vi "test26-MappingRelationshipByLocalRegistration_WithSubcriberName.vi"(8 "error in (no error)":errorcluster, 11 "TestCase in":refnum<class "testcase-CSMBroadcast.lvclass">) -> (0 "error out":errorcluster, 3 "TestCase out":refnum<class "testcase-CSMBroadcast.lvclass">)   [LabVIEW 2017, in "testcase-CSMBroadcast.lvclass"]
uses:
  testcase-CSMBroadcast.lvclass
  caa41fc0-4920-4570-a7eb-0567c3b7bd6c.vi
  <vilib>/addons/_JKI Toolkits/VI Tester/TestCase.llb/TestCase.lvclass
  src/user.lib/_NEVSTOP/Communicable State Machine(CSM)/Communicable State Machine.lvlib
  C:/Program Files (x86)/National Instruments/LabVIEW 2017/vi.lib/addons/_JKI Toolkits/VI Tester/TestCase.llb/TestCase.lvclass
panel:
  out "Loop Count":i32
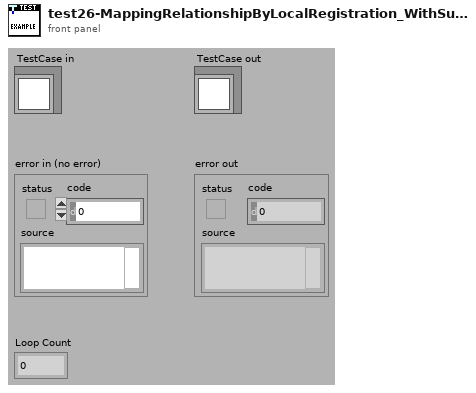
[diagram p1: front panel]
types:
  T1 = cluster{"Status":string, "Source CSM":string, "Target CSM":string, "Target API":string}[]
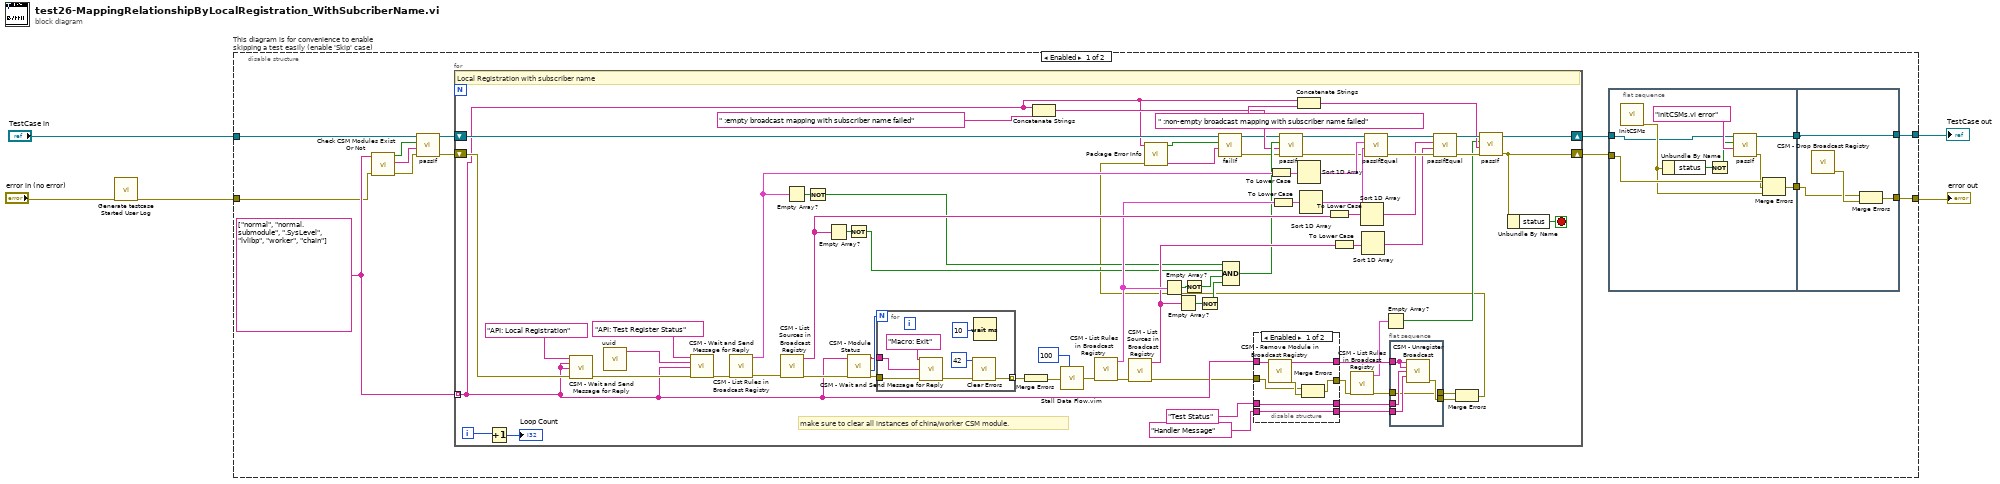
[diagram p0: block diagram]
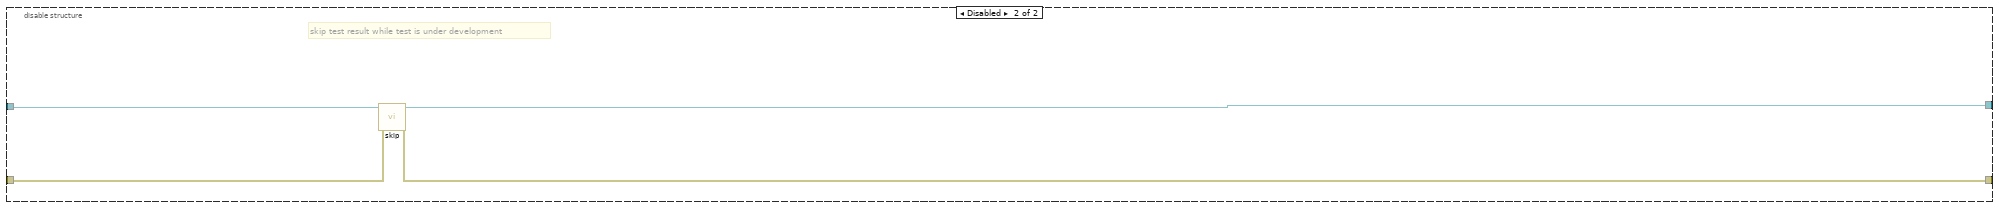
[diagram p3: hidden frame]
diagram:
  n1 = call "Generate testcase Started User Log.vi"("Error In"="error in (no error)") -> ("error out"=w1:errorcluster)  [unwired: 10 in]
  n2 = disable-structure "This diagram is for convenience to enable skipping a test easily (enable 'Skip' case)" shown="Enabled" {
    disable-tunnel: "TestCase in" -> [w15 w130]
    disable-tunnel: [w7 w128] -> w2
    disable-tunnel: [w6 w129] -> w4
    disable-tunnel: w1 -> [w13 w127]
    frame Enabled {
      w16 = string[] ["normal", "normal.submodule", ".SysLevel", "lvlibp", "worker", "chain"]
      n3 = call "Check CSM Modules Exist Or Not.vi"("error in"=w13, "CSM names in"=w16) -> ("error out"=w17:errorcluster, "Debug string"=w18:string, "All Modules Exist?"=w19:bool)  [unwired: 7 in]
      n4 = call-dynamic "passIf.vi"("error in (no error)"=w17, "message (\"\")"=w18, "pass"=w19, "TestCase in"=w15) -> ("error out"=w12:errorcluster, "TestCase out"=w14:refnum<class "testcase-CSMBroadcast.lvclass">)  [unwired: 6 in]
      n5 = for {
        tunnel: w16 -> [w39] mode=indexing
        shift-right: [w69] -> w9
        shift-left: w14 -> [w50]
        shift-right: [w70] -> w8
        shift-left: w12 -> [w60]
        i -> [w84]
        stop <- w97 stop-if-true
        # "make sure to clear all instances of china/worker CSM module."
        # "Local Registration with subscriber name"
        n6 = Increment(x=w84) -> (x+1=→"Loop Count":i32)
        n7 = call "CSM - Wait and Send Message for Reply.vi"("State"="API: Local Registration", "Arguments (\"\")"=w39, "Target Module"=w39, "Error In (No Error)"=w60) -> ("error out"=w102:errorcluster)  [unwired: 8 in, 3 out]
        n8 = call "uuid.vi"() -> ("UUID"=w100:string)  [unwired: 11 in]
        n9 = call "CSM - Wait and Send Message for Reply.vi"("State"="API: Test Register Status", "Arguments (\"\")"=w100, "Target Module"=w39, "Error In (No Error)"=w102) -> ("error out"=w99:errorcluster)  [unwired: 8 in, 3 out]
        n10 = call "CSM - List Rules in Broadcast Registry.vi"("error in (no error)"=w99) -> ("error out"=w96:errorcluster, "Rule Entries"=w82:T1)  [unwired: 8 in, 1 out]
        n11 = call "CSM - List Sources in Broadcast Registry.vi"("error in (no error)"=w96) -> ("error out"=w65:errorcluster, "Broadcast Names"=w79:string[])  [unwired: 9 in]
        n12 = Empty Array?(array=w82) -> (empty?=w81:bool)
        n13 = Not(x=w81) -> (.not. x?=w74:bool)
        n14 = Empty Array?(array=w79) -> (empty?=w80:bool)
        n15 = Not(x=w80) -> (.not. x?=w73:bool)
        n16 = call "CSM - Module Status.vi"("Error In"=w65, "CSM Name"=w39) -> ("error out"=w66:errorcluster, "#Nodes"=w68:i32, "CSM Name (Dup)"=w67:string)  [unwired: 5 in, 2 out]
        n17 = for {
          N: w68 -> [_]
          tunnel: w67 -> [w125]
          tunnel: w66 -> [w124]
          tunnel: [w122] -> w98 mode=indexing
          n18 = call "CSM - Wait and Send Message for Reply.vi"("State"="Macro: Exit", "Target Module"=w125, "Error In (No Error)"=w124) -> ("error out"=w123:errorcluster)  [unwired: 9 in, 3 out]
          n19 = call <vilib>:"Clear Errors.vi"("error in (no error)"=w123, "specific error code to clear (0: all)"=42) -> ("error out"=w122:errorcluster)  [unwired: 4 in, 1 out]
          n20 = Wait (ms)(milliseconds to wait=u32 10) -> ()  [unwired: 1 out]
        }
        n21 = Merge Errors(w98) -> (w54:errorcluster)
        n22 = Concatenate Strings(w39, " :empty broadcast mapping with subscriber name failed" ("string")) -> (w56:string)
        n23 = call "Stall Data Flow.vim"("value in"=w54, "milliseconds to wait"=u32 100) -> ("value out"=w53:errorcluster)  [unwired: 1 out]
        n24 = call "CSM - List Rules in Broadcast Registry.vi"("error in (no error)"=w53) -> ("error out"=w95:errorcluster, "Rule Entries"=w77:T1)  [unwired: 8 in, 1 out]
        n25 = call "CSM - List Sources in Broadcast Registry.vi"("error in (no error)"=w95) -> ("error out"=w38:errorcluster, "Broadcast Names"=w75:string[])  [unwired: 9 in]
        n26 = Empty Array?(array=w77) -> (empty?=w78:bool)
        n27 = Empty Array?(array=w75) -> (empty?=w76:bool)
        n28 = Not(x=w78) -> (.not. x?=w72:bool)
        n29 = Not(x=w76) -> (.not. x?=w71:bool)
        n30 = Compound Arithmetic op=AND(w74, w73, w72, w71) -> (w59:bool)
        n31 = disable-structure shown="Enabled" {
          disable-tunnel: w38 -> [w109 w118]
          disable-tunnel: [w113 w118] -> w45
          disable-tunnel: w39 -> [w114 w119]
          disable-tunnel: "Test Status" ("Status") -> [w111 w117]
          disable-tunnel: "Handler Message" ("Response Message (If \"\", Same as Source Message)") -> [w110 w116]
          disable-tunnel: [w112 w119] -> w46
          disable-tunnel: [w111 w117] -> w44
          disable-tunnel: [w110 w116] -> w43
          frame Enabled {
            n32 = call "CSM - Remove Module in Broadcast Registry.vi"("CSM Name"=w114) -> ("CSM Name (Dup)"=w112:string, "error out"=w115:errorcluster)  [unwired: 13 in]
            n33 = Merge Errors(w109, w115) -> (w113:errorcluster)
          }
          frame Disabled {
          }
        }
        n34 = To Lower Case(string=w82) -> (all lower case string=w94:T1)
        n35 = To Lower Case(string=w77) -> (all lower case string=w93:T1)
        n36 = Concatenate Strings(w39, " :non-empty broadcast mapping with subscriber name failed" ("string")) -> (w55:string)
        n37 = Sort 1D Array(array=w94) -> (sorted array=w92:T1)
        n38 = Sort 1D Array(array=w93) -> (sorted array=w91:T1)
        n39 = To Lower Case(string=w79) -> (all lower case string=w88:string[])
        n40 = To Lower Case(string=w75) -> (all lower case string=w87:string[])
        n41 = call "CSM - List Rules in Broadcast Registry.vi"("error in (no error)"=w45) -> ("error out"=w41:errorcluster, "Rule Entries"=w35:T1)  [unwired: 8 in, 1 out]
        n42 = Sort 1D Array(array=w88) -> (sorted array=w86:string[])
        n43 = Sort 1D Array(array=w87) -> (sorted array=w85:string[])
        n44 = Empty Array?(array=w35) -> (empty?=w34:bool)
        n45 = flat-sequence {
          tunnel: w46 -> [w108]
          tunnel: w44 -> [w107]
          tunnel: w43 -> [w106]
          tunnel: [w105] -> w42
          tunnel: w41 -> [w104]
          tunnel: [w104] -> w40
          frame #0 {
            n46 = call "CSM - Unregister Broadcast.vi"("CSM Name(Empty for Broadcast Event)"=w108, "Source CSM Name (* as Default)"=w108, "Trigger"=w107, "API (\"*\" as Default)"=w106) -> ("error out"=w105:errorcluster)  [unwired: 10 in, 1 out]
          }
        }
        n47 = Merge Errors(w40, w42) -> (w33:errorcluster)
        n48 = call "Package Error Info.vi"("error in"=w33, "String in"=w39) -> ("packed error info out"=w47:string, "error status"=w48:bool)  [unwired: 8 in]
        n49 = call-dynamic "failIf.vi"("message (\"\")"=w47, "fail"=w48, "TestCase in"=w50) -> ("error out"=w49:errorcluster, "TestCase out"=w51:refnum<class "testcase-CSMBroadcast.lvclass">)  [unwired: 7 in]
        n50 = call-dynamic "passIf.vi"("error in (no error)"=w49, "message (\"\")"=w56, "pass"=w59, "TestCase in"=w51) -> ("error out"=w61:errorcluster, "TestCase out"=w62:refnum<class "testcase-CSMBroadcast.lvclass">)  [unwired: 6 in]
        n51 = call-dynamic "passIfEqual.vi"("error in (no error)"=w61, "y"=w91, "x"=w92, "TestCase in"=w62) -> ("error out"=w89:errorcluster, "TestCase out"=w90:refnum<class "testcase-CSMBroadcast.lvclass">)  [unwired: 6 in]
        n52 = call-dynamic "passIfEqual.vi"("error in (no error)"=w89, "y"=w85, "x"=w86, "TestCase in"=w90) -> ("error out"=w63:errorcluster, "TestCase out"=w64:refnum<class "testcase-CSMBroadcast.lvclass">)  [unwired: 6 in]
        n53 = call-dynamic "passIf.vi"("error in (no error)"=w63, "message (\"\")"=w55, "pass"=w34, "TestCase in"=w64) -> ("error out"=w70:errorcluster, "TestCase out"=w69:refnum<class "testcase-CSMBroadcast.lvclass">)  [unwired: 6 in]
        n54 = Unbundle By Name(w70) -> ("status"=w97:bool)
      }
      n55 = flat-sequence {
        tunnel: w9 -> [w20]
        tunnel: [w28] -> w11
        tunnel: w8 -> [w25]
        tunnel: [w22] -> w10
        tunnel: w11 -> [w31]
        tunnel: [w31] -> w7
        tunnel: [w30] -> w6
        tunnel: w10 -> [w29]
        frame #0 {
          n56 = call "InitCSMs.vi"() -> ("error out"=w23:errorcluster)  [unwired: 10 in, 1 out]
          n57 = Unbundle By Name(w23) -> ("status"=w27:bool)
          n58 = Not(x=w27) -> (.not. x?=w21:bool)
          n59 = call-dynamic "passIf.vi"("message (\"\")"="initCSMs.vi error" ("message (\"\")"), "pass"=w21, "TestCase in"=w20) -> ("error out"=w24:errorcluster, "TestCase out"=w28:refnum<class "testcase-CSMBroadcast.lvclass">)  [unwired: 7 in]
          n60 = Merge Errors(w25, w24, w23) -> (w22:errorcluster)
        }
        frame #1 {
          n61 = call "CSM - Drop Broadcast Registry.vi"() -> ("error out"=w32:errorcluster)  [unwired: 15 in]
          n62 = Merge Errors(w29, w32) -> (w30:errorcluster)
        }
      }
    }
    frame Disabled {
      # "skip test result while test is under development"
      n63 = call <vilib>:"skip.vi"("error in (no error)"=w127, "TestCase in"=w130) -> ("error out"=w129:errorcluster, "TestCase out"=w128:refnum<class "testcase-CSMBroadcast.lvclass">)  [unwired: 8 in]
    }
  }
  "error out" <- w4
  "TestCase out" <- w2
